vi "test.vi"   [LabVIEW 2013]
uses:
  <vilib>/robotics/Obstacle Avoidance/Simple Vector Field Histogram/NI_Robotics_Simple Vector Field Histogram.lvlib
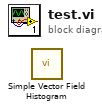
[diagram p0: block diagram]
diagram:
  n1 = call <vilib>:"Simple Vector Field Histogram.vi"() -> ()  [unwired: 7 in, 5 out]
